vi "Convert Velocity To Acceleration.vi"(8 "loopTime":dbl, 9 "driveCountsPerInch":dbl, 11 "velocity:  ticks/100 ms":dbl) -> (3 "m / s^2":dbl)   [LabVIEW 2020]
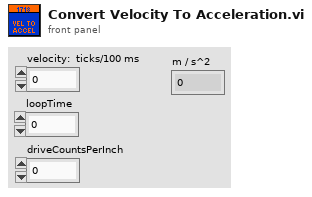
[diagram p1: front panel]
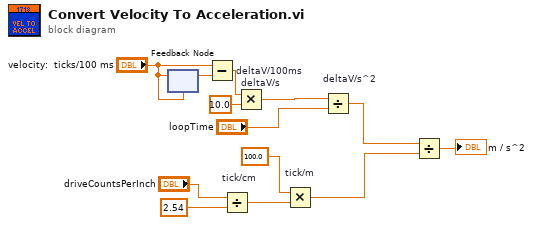
[diagram p0: block diagram]
diagram:
  n1 = feedback #1("velocity:  ticks/100 ms") -> (w10:dbl)
  n2 = feedback-in #1("velocity:  ticks/100 ms") -> ()
  n3 = Subtract "deltaV/100ms"(x="velocity:  ticks/100 ms", y=w10) -> (x-y=w8:dbl)
  n4 = Divide "tick/cm"(x="driveCountsPerInch", y=2.54) -> (x/y=w6:dbl)
  n5 = Multiply "deltaV/s"(x=w8, y=10.0) -> (x*y=w13:dbl)
  n6 = Multiply "tick/m"(x=100.0, y=w6) -> (x*y=w4:dbl)
  n7 = Divide "deltaV/s^2"(x=w13, y="loopTime") -> (x/y=w3:dbl)
  n8 = Divide(x=w3, y=w4) -> (x/y=→"m / s^2":dbl)
